vi "DroneVideoAndData.vi"() -> ()   [LabVIEW 2017]
uses:
  <vilib>/LVH/AR Drone Toolkit/AR Drone.lvlib
  <vilib>/LVH/AR Drone Toolkit/Decode NavData/Typedefs/NavData Demo.ctl
panel:
  out "Video Stream":picture
  out "NavData Out":T1
  out "Battery Remaining":dbl(slide) scale=0.0..100.0
  in  "Hover":bool
  in  "Take Off/Land":bool
  in  "Emergency Landing":bool
  in  "stop":bool
  in  "Control Cluster":T2 {"Yaw Speed" scale=-1.0..1.0; "Vertical Speed" scale=-1.0..1.0; "Pitch" scale=-1.0..1.0; "Roll" scale=-1.0..1.0}
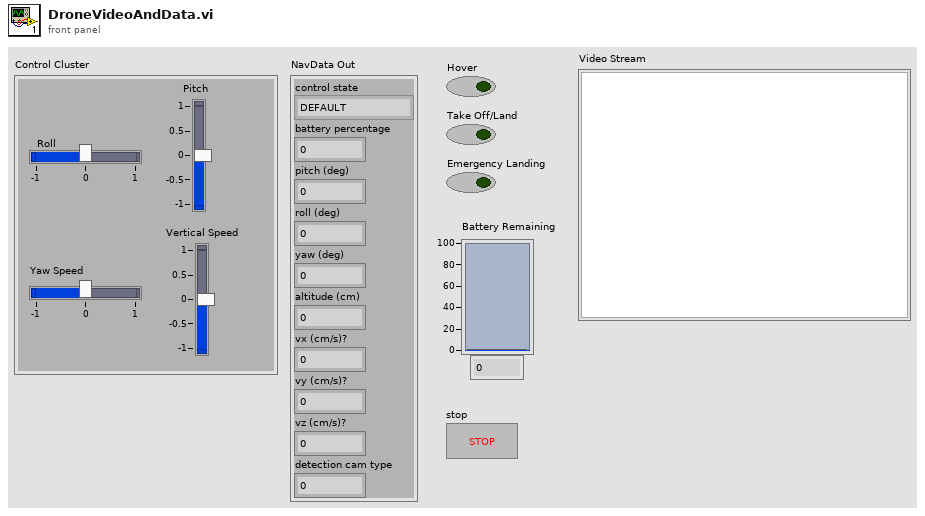
[diagram p1: front panel]
types:
  T1 = typedef "AR Drone.lvlib/NavData Demo.ctl" = cluster{"control state":enum32{"DEFAULT", "INIT", "LANDING", "FLYING", "HOVERING", "TEST", "TRANS_TAKEOFF", "TRANS_GOTOFIX", "TRANS_LANDING"}, "battery percentage":u32, "pitch (deg)":sgl, "roll (deg)":sgl, "yaw (deg)":sgl, "altitude (cm)":u32, "vx (cm/s)?":sgl, "vy (cm/s)?":sgl, "vz (cm/s)?":sgl, "detection cam type":u32}
  T2 = cluster{"Roll":sgl, "Pitch":sgl, "Vertical Speed":sgl, "Yaw Speed":sgl}
  T3 = typedef "AR Drone.lvlib/AR Drone Resource.ctl" = cluster{"UDP Control Connection":refnum<k16>, "UDP NavData Connection":refnum<k16>, "UDP Video Connection (Drone 1.0)":refnum<k16>, "TCP Video Connection (Drone 2.0)":refnum<k5>, "TCP Control Port Connection":refnum<k5>, "Drone IP address":string, "Drone Command Port":u16, "Drone NavData Port":u16, "Drone Vid Stream Port":u16, "Drone TCP Control Port":u16, "Home IP address":string, "Home Command Port":u16, "Home NavData Port":u16, "Home Vid Stream Port":u16, "Drone Version":i32}
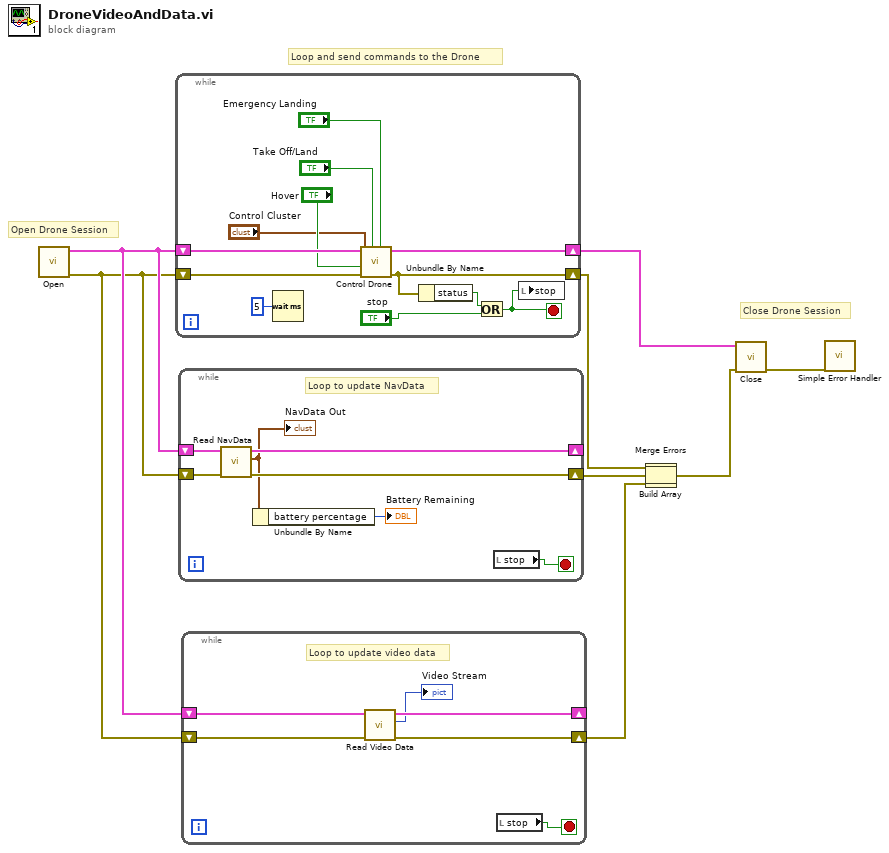
[diagram p0: block diagram]
diagram:
  # "Close Drone Session"
  # "Loop and send commands to the Drone"
  # "Open Drone Session"
  n1 = call <vilib>:"Open.vi"() -> ("error out"=w3:errorcluster, "AR Drone Resource"=w4:T3)  [unwired: 10 in]
  n2 = while {
    shift-right: [w16] -> w9
    shift-left: w4 -> [w20]
    shift-right: [w11] -> w7
    shift-left: w3 -> [w21]
    stop <- w10 stop-if-true
    n3 = Wait (ms)(milliseconds to wait=u32 5) -> ()  [unwired: 1 out]
    n4 = call <vilib>:"Control Drone.vi"("Emergency Landing"="Emergency Landing", "Takeoff/Land"="Take Off/Land", "error in (no error)"=w21, "Hover"="Hover", "Control Cluster"="Control Cluster", "AR Drone Resource"=w20) -> ("error out"=w11:errorcluster, "AR Drone Resource Out"=w16:T3)  [unwired: 4 in]
    n5 = Unbundle By Name(w11) -> ("status"=w13:bool)
    n6 = Or(x=w13, y="stop") -> (x .or. y?=w10:bool)
    n7 = local write "stop"(w10) -> ()
  }
  n8 = while {
    shift-right: [w26] -> _
    shift-left: w4 -> [w27]
    shift-right: [w24] -> w8
    shift-left: w3 -> [w25]
    stop <- w28 stop-if-true
    # "Loop to update NavData"
    n9 = call <vilib>:"Read NavData.vi"("error in (no error)"=w25, "AR Drone Resource"=w27) -> ("error out"=w24:errorcluster, "NavData Out"=w23:T1, "AR Drone Resource Out"=w26:T3)  [unwired: 7 in]
    "NavData Out" <- w23
    n10 = Unbundle By Name(w23) -> ("battery percentage"=→"Battery Remaining":u32)
    n11 = local read "stop"() -> (w28:bool)
  }
  n12 = while {
    shift-right: [w31] -> _
    shift-left: w4 -> [w33]
    shift-right: [w30] -> w2
    shift-left: w3 -> [w32]
    stop <- w34 stop-if-true
    # "Loop to update video data"
    n13 = call <vilib>:"Read Video Data.vi"("error in (no error)"=w32, "AR Drone Resource"=w33) -> ("error out"=w30:errorcluster, "Video Stream"=→"Video Stream":picture, "AR Drone Resource Out"=w31:T3)  [unwired: 7 in]
    n14 = local read "stop"() -> (w34:bool)
  }
  n15 = Build Array(w7, w8, w2) -> (w5:errorcluster[])
  n16 = Merge Errors(w5) -> (w1:errorcluster)  [unwired: 1 in]
  n17 = call <vilib>:"Close.vi"("error in (no error)"=w1, "AR Drone Resource"=w9) -> ("error out"=w6:errorcluster)  [unwired: 9 in]
  n18 = call <vilib>:"Simple Error Handler.vi"("error in (no error)"=w6) -> ()  [unwired: 4 in, 5 out]
